vi "Compare to the Cent.vi"(4 "Dollar y":dbl, 5 "Dollar x":dbl) -> (2 "x = y?":bool)   [LabVIEW 2018]
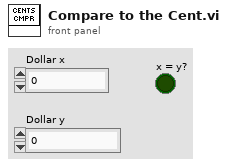
[diagram p1: front panel]
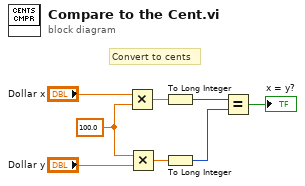
[diagram p0: block diagram]
diagram:
  w6 = 100.0 ("y")
  # "Convert to cents"
  n1 = Multiply(x="Dollar x", y=w6) -> (x*y=w5:dbl)
  n2 = Multiply(x=w6, y="Dollar y") -> (x*y=w4:dbl)
  n3 = To Long Integer(number=w5) -> (32bit integer=w3:i32)
  n4 = To Long Integer(number=w4) -> (32bit integer=w2:i32)
  n5 = Equal?(x=w3, y=w2) -> (x = y?=→"x = y?":bool)
